vi "Destruct.vi"(8 "error in (no error)":errorcluster, 11 "muExpr in":refnum<class "muExpr.lvclass">) -> (0 "error out":errorcluster)   [LabVIEW 2015, in "muParser.lvlib" / "muExpr.lvclass"]
uses:
  muExpr.lvclass
  muExpr.lvclass/muExpr.ctl
  muParser.lvlib
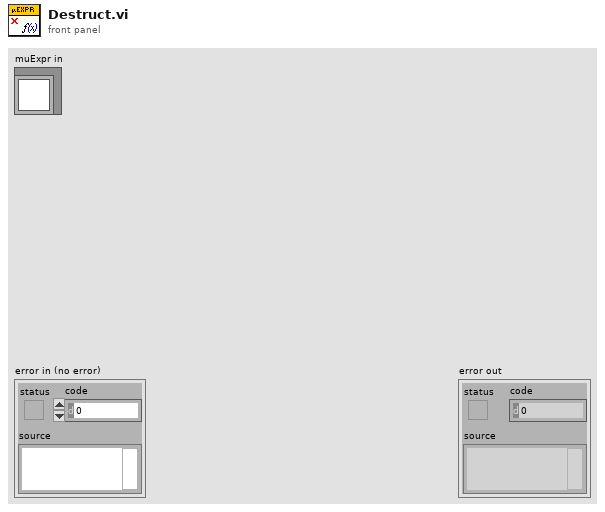
[diagram p1: front panel]
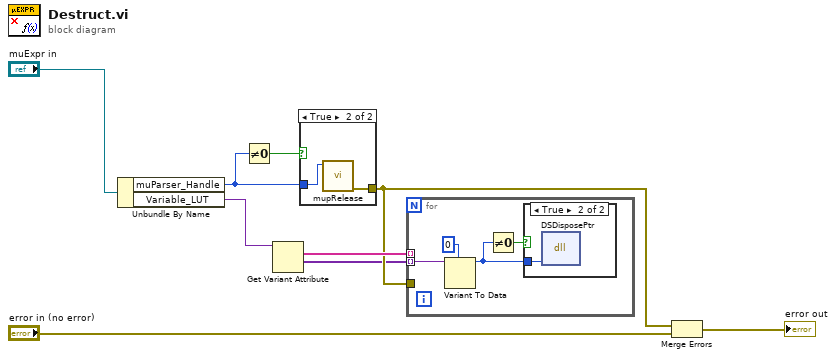
[diagram p0: block diagram]
diagram:
  n1 = Unbundle By Name("muExpr in") -> ("muParser_Handle"=w2:u64, "Variable_LUT"=w6:variant)
  n2 = Not Equal To 0?(x=w2) -> (x != 0?=w1:bool)
  n3 = Get Variant Attribute(Variant=w6) -> (names=w5:string[], values=w3:variant[])  [unwired: 3 in, 2 out]
  n4 = case shown="True" w1 {
    tunnel: [_ w10] -> w4
    tunnel: w2 -> [_ w11]
    frame False {
    }
    frame True {
      n5 = call "mupRelease.vi"("hParser"=w11) -> ("error out"=w10:errorcluster)  [unwired: 10 in]
    }
  }
  n6 = for {
    tunnel: w5 -> [_] mode=indexing
    tunnel: w4 -> [_]
    tunnel: w3 -> [w15] mode=indexing
    n7 = Variant To Data(type=u64 0, Variant=w15) -> (data=w13:u64)  [unwired: 1 in, 1 out]
    n8 = Not Equal To 0?(x=w13) -> (x != 0?=w12:bool)
    n9 = case shown="True" w12 {
      tunnel: w13 -> [_ w16]
      frame False {
      }
      frame True {
        n10 = dll-call lib="LabVIEW" fn="DSDisposePtr"("ptr"=w16) -> ()  [unwired: 5 in, 2 out]
      }
    }
  }
  n11 = Merge Errors(w4, "error in (no error)") -> (→"error out":errorcluster)
